vi "Finalize View Init.vi"(8 "error in (no error)":errorcluster, 10 "View Name":string, 11 "Example Controller Actor in":refnum<class "Example Controller.lvclass">) -> (0 "error out":errorcluster, 3 "Example Controller Actor out":refnum<class "Example Controller.lvclass">)   [LabVIEW 2023, in "Example GUI View.lvlib" / "Example Controller.lvclass"]
uses:
  Example Controller.lvclass
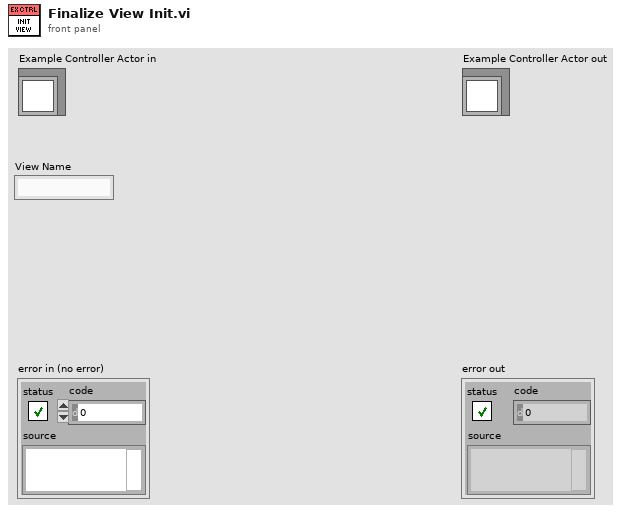
[diagram p1: front panel]
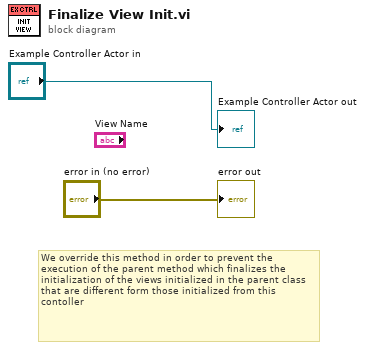
[diagram p0: block diagram]
diagram:
  # "We override this method in order to prevent the execution of the parent method which finalizes the initialization of the views initialized in the parent class that are different form those initialized from this contoller"
  "error out" <- "error in (no error)"
  "Example Controller Actor out" <- "Example Controller Actor in"
